vi "Read UDVs.vi"(7 "R/W Case":T1, 8 "error in (no error)":errorcluster, 9 "Output FIFO buffer in":dbl[](array[numeric]), 10 "Output Data in":T6 {"BD Refs"."Data Reference" format="%.0x"}, 11 "UDVs in":T2[](array[typedef]) {"VS ref" format="%.0x"}) -> (0 "error out":errorcluster, 1 "Output FIFO buffer out":dbl[](array[numeric]), 2 "Output Data out":T6 {"BD Refs"."Data Reference" format="%.0x"}, 3 "UDVs out":T2[](array[typedef]) {"VS ref" format="%.0x"})   [LabVIEW 2016, in "Scan Engine Custom Device.lvlib"]
uses:
  Scan Engine Custom Device.lvlib
  Type Defs/Output Data.ctl
  <vilib>/NI Veristand/Custom Device API/Block Data Reference.ctl
  <vilib>/NI Veristand/Custom Device API/Data Reference.ctl
  Type Defs/UDV Data.ctl
  <vilib>/NI Veristand/Custom Device API/Custom Device Item Ref.ctl
  Type Defs/UDV Data Type.ctl
  Type Defs/FXP Config.ctl
  Type Defs/RW Case.ctl
  <vilib>/NI Veristand/Custom Device API/Global Data Refs.vi
  <vilib>/NI Veristand/Custom Device API/Custom Device API.lvlib
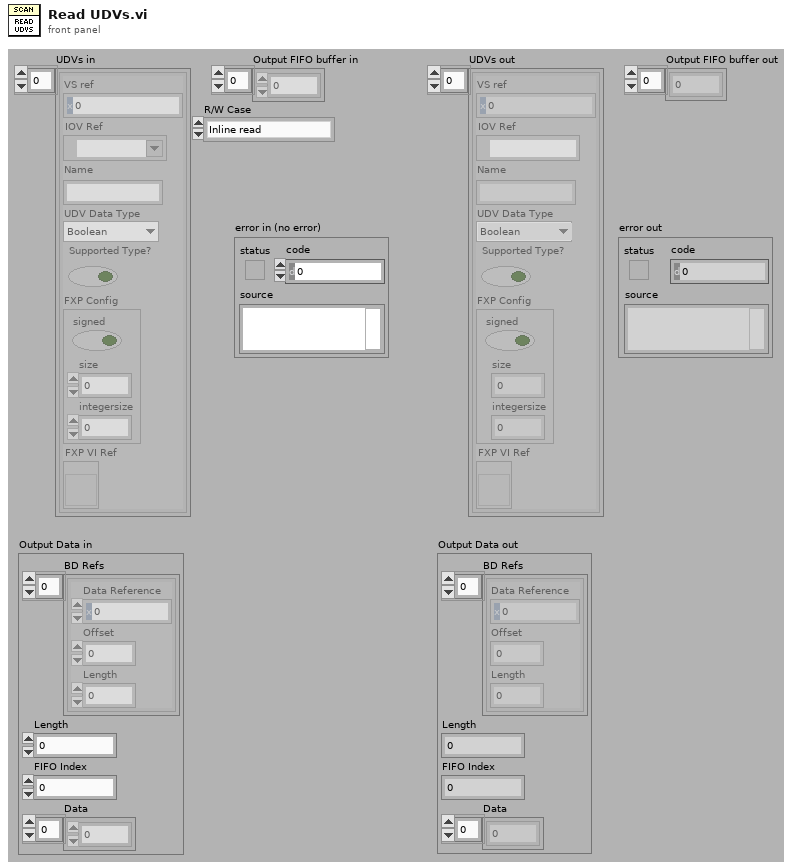
[diagram p1: front panel]
types:
  T1 = typedef "Scan Engine Custom Device.lvlib/RW Case.ctl" = enum16{"Inline read", "Inline write", "Async - Inline loop read", "Async - Inline loop write", "Async loop (read/write)"}
  T2 = typedef "Scan Engine Custom Device.lvlib/UDV Data.ctl" = cluster{"VS ref":T3, "IOV Ref":refnum<k21>, "Name":string, "UDV Data Type":T4, "Supported Type?":bool, "FXP Config":T5, "FXP VI Ref":refnum<vi>}
  T3 = typedef "Custom Device API.lvlib/Custom Device Item Ref.ctl" = u64
  T4 = typedef "Scan Engine Custom Device.lvlib/UDV Data Type.ctl" = enum16{"Boolean", "Fixed Point", "Int8", "Int16", "Int32", "Int64", "U32 Bit Field", "UInt8", "UInt16", "UInt32", "UInt64", "Other"}
  T5 = typedef "Scan Engine Custom Device.lvlib/FXP Config.ctl" = cluster{"signed":bool, "size":u32, "integersize":i32}
  T6 = typedef "Scan Engine Custom Device.lvlib/Output Data.ctl" = cluster{"BD Refs":T7[], "Length":i32, "FIFO Index":i32, "Data":dbl[]}
  T7 = typedef "Custom Device API.lvlib/Block Data Reference.ctl" = cluster{"Data Reference":T8, "Offset":u64, "Length":u64}
  T8 = typedef "Custom Device API.lvlib/Data Reference.ctl" = i32
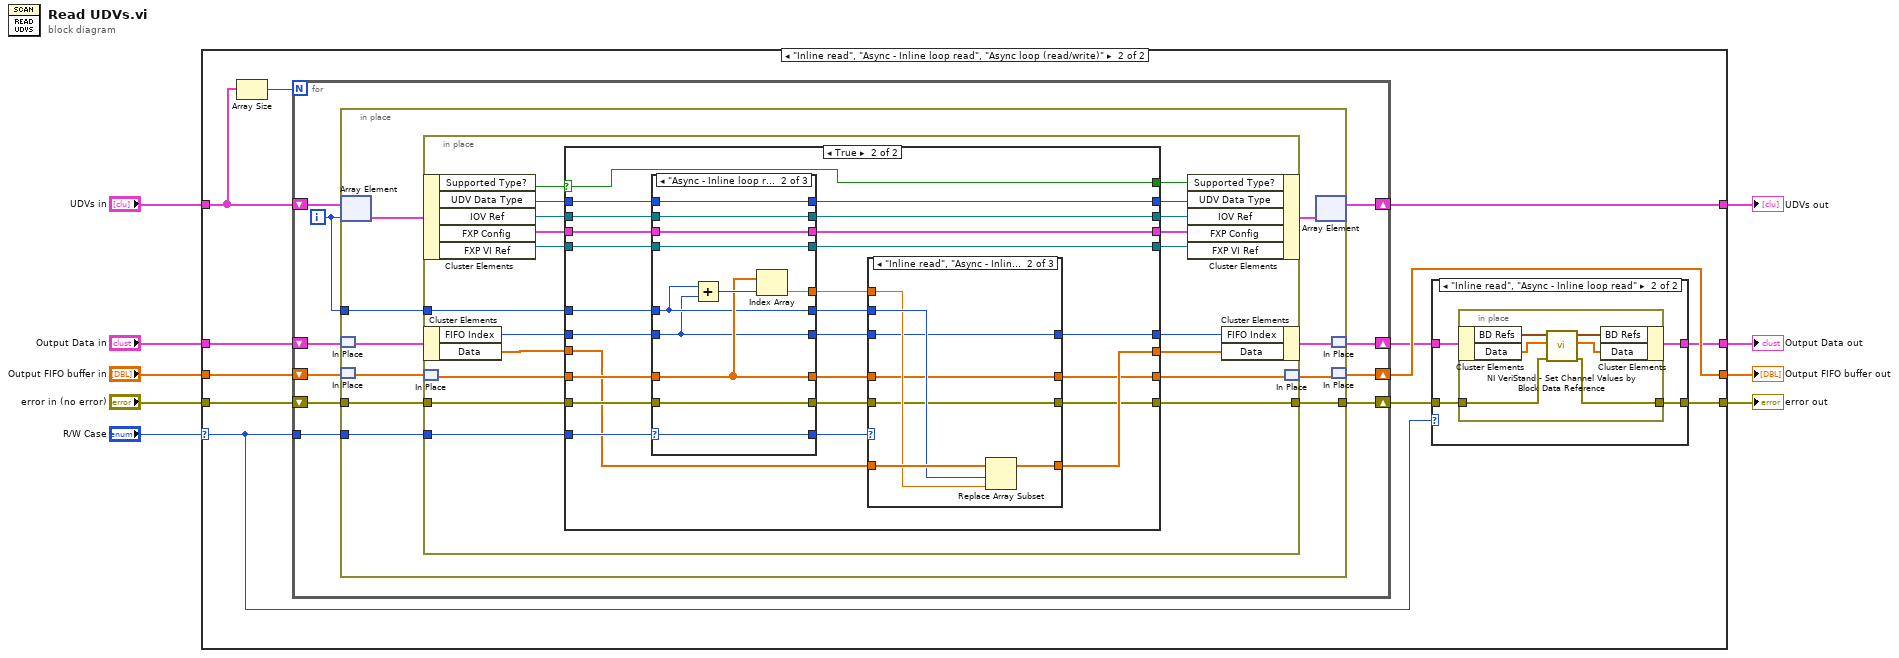
[diagram p0: block diagram]
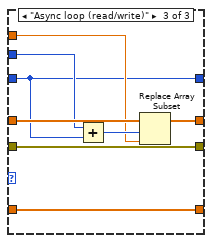
[diagram p5: hidden frame]
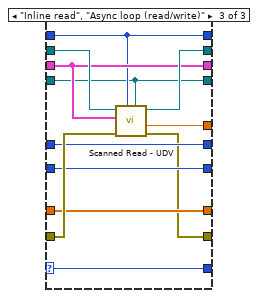
[diagram p7: hidden frame]
diagram:
  n1 = case shown="\"Inline read\", \"Async - Inline loop read\", \"Async loop (read/write)\"" "R/W Case" {
    selector: "R/W Case" -> [_ w14]
    tunnel: [w11 w25] -> w2
    tunnel: "Output FIFO buffer in" -> [w11 w24]
    tunnel: [w12 w16] -> w9
    tunnel: [w13 w23] -> w8
    tunnel: "Output Data in" -> [w12 w22]
    tunnel: "UDVs in" -> [w13 w21]
    tunnel: [w10 w15] -> w5
    tunnel: "error in (no error)" -> [w10 w19]
    frame Default {
    }
    frame "Inline read", "Async - Inline loop read", "Async loop (read/write)" {
      n2 = Array Size(array=w21) -> (size(s)=w20:i32)
      n3 = for {
        N: w20 -> [_]
        shift-right: [w34] -> w23
        shift-left: w21 -> [w35]
        shift-right: [w26] -> w18
        shift-left: w22 -> [w29]
        shift-right: [w32] -> w25
        shift-left: w24 -> [w33]
        shift-right: [w30] -> w17
        shift-left: w19 -> [w31]
        tunnel: w14 -> [w28]
        i -> [w27]
        n4 = in-place {
          in-place-border: w31 -> [w42]
          in-place-border: [w36] -> w30
          in-place-border: w28 -> [w41]
          in-place-border: w27 -> [w40]
          n5 = in-place-array #1(w35, w27) -> (w45:T2)
          n6 = in-place-match #2(w29) -> (w44:T6)
          n7 = in-place-match #3(w33) -> (w43:dbl[])
          n8 = in-place {
            in-place-border: w42 -> [w58]
            in-place-border: w41 -> [w46]
            in-place-border: w40 -> [w59]
            in-place-border: [w52] -> w36
            n9 = in-place-cluster #4(w45) -> ("Supported Type?"=w65:bool, "UDV Data Type"=w61:T4, "IOV Ref"=w60:refnum<k21>, "FXP Config"=w64:T5, "FXP VI Ref"=w63:refnum<vi>)
            n10 = in-place-cluster #5(w44) -> ("FIFO Index"=w50:i32, "Data"=w62:dbl[])
            n11 = in-place-match #6(w43) -> (w49:dbl[])
            n12 = case shown="True" w65 {
              selector: w65 -> [w73 w90]
              tunnel: w64 -> [w70 w96]
              tunnel: w63 -> [w69 w95]
              tunnel: w50 -> [w68 w94]
              tunnel: w62 -> [w67 w79]
              tunnel: w46 -> [_ w99]
              tunnel: w61 -> [w72 w98]
              tunnel: w60 -> [w71 w97]
              tunnel: w49 -> [w66 w93]
              tunnel: w59 -> [_ w92]
              tunnel: w58 -> [w74 w91]
              tunnel: [w73 w90] -> w57
              tunnel: [w72 w89] -> w56
              tunnel: [w71 w88] -> w55
              tunnel: [w70 w87] -> w54
              tunnel: [w69 w86] -> w53
              tunnel: [w74 w76] -> w52
              tunnel: [w68 w78] -> w47
              tunnel: [w67 w77] -> w51
              tunnel: [w66 w75] -> w48
              frame False {
              }
              frame True {
                n13 = case shown="\"Async - Inline loop read\"" w99 {
                  selector: w99 -> [w119 w133 w141]
                  tunnel: w98 -> [w120 w131 w142]
                  tunnel: w97 -> [w121 w132 w150]
                  tunnel: w96 -> [w122 w130 w148]
                  tunnel: w95 -> [w123 w129 w140]
                  tunnel: w94 -> [w125 w134 w145]
                  tunnel: w93 -> [w126 w137 w144]
                  tunnel: [w126 w137 w144] -> w81
                  tunnel: w92 -> [w124 w135 w146]
                  tunnel: [_ w136 w139] -> w82
                  tunnel: [w124 w135 w146] -> w84
                  tunnel: [w125 w134 w145] -> w83
                  tunnel: [w119 w133 w141] -> w85
                  tunnel: [w121 w132 w149] -> w88
                  tunnel: [w120 w131 w142] -> w89
                  tunnel: [w122 w130 w148] -> w87
                  tunnel: [w123 w129 w140] -> w86
                  tunnel: w91 -> [w127 w128 w147]
                  tunnel: [w127 w128 w143] -> w80
                  frame Default {
                  }
                  frame "Async - Inline loop read" {
                    n14 = Add(x=w135, y=w134) -> (x+y=w138:i32)
                    n15 = Index Array(array=w137, index=w138) -> (element=w136:dbl)
                  }
                  frame "Inline read", "Async loop (read/write)" {
                    n16 = call "Scanned Read - UDV.vi"("FXP VI Ref"=w140, "UDV Data Type"=w142, "error in (no error)"=w147, "FXP Config"=w148, "IOV ref in"=w150) -> ("error out"=w143:errorcluster, "data out"=w139:dbl, "IOV ref out"=w149:refnum<k21>)  [unwired: 4 in]
                  }
                }
                n17 = case shown="\"Inline read\", \"Async - Inline loop read\"" w85 {
                  tunnel: w84 -> [_ w109 w117]
                  tunnel: w83 -> [w103 w104 w111]
                  tunnel: w82 -> [_ w108 w115]
                  tunnel: w81 -> [w100 w105 w118]
                  tunnel: w80 -> [w101 w106 w113]
                  tunnel: w79 -> [w102 w110 w112]
                  tunnel: [w103 w104 w111] -> w78
                  tunnel: [w102 w107 w112] -> w77
                  tunnel: [w101 w106 w113] -> w76
                  tunnel: [w100 w105 w114] -> w75
                  frame Default {
                  }
                  frame "Inline read", "Async - Inline loop read" {
                    n18 = Replace Array Subset(array=w110, new element=w108, index=w109) -> (w107:dbl[])
                  }
                  frame "Async loop (read/write)" {
                    n19 = Add(x=w117, y=w111) -> (x+y=w116:i32)
                    n20 = Replace Array Subset(array=w118, new element=w115, index=w116) -> (w114:dbl[])
                  }
                }
              }
            }
            n21 = in-place-cluster #4("Supported Type?"=w57, "UDV Data Type"=w56, "IOV Ref"=w55, "FXP Config"=w54, "FXP VI Ref"=w53) -> (w39:T2)
            n22 = in-place-cluster #5("FIFO Index"=w47, "Data"=w51) -> (w38:T6)
            n23 = in-place-match #6(w48) -> (w37:dbl[])
          }
          n24 = in-place-array #1(w39) -> (w34:T2[])  [unwired: 1 out]
          n25 = in-place-match #2(w38) -> (w26:T6)
          n26 = in-place-match #3(w37) -> (w32:dbl[])
        }
      }
      n27 = case shown="\"Inline read\", \"Async - Inline loop read\"" w14 {
        tunnel: w18 -> [w151 w156]
        tunnel: w17 -> [w152 w155]
        tunnel: [w152 w154] -> w15
        tunnel: [w151 w153] -> w16
        frame Default {
        }
        frame "Inline read", "Async - Inline loop read" {
          n28 = in-place {
            in-place-border: w155 -> [w158]
            in-place-border: [w157] -> w154
            n29 = in-place-cluster #7(w156) -> ("BD Refs"=w162:T7[], "Data"=w160:dbl[])
            n30 = call <vilib>:"NI VeriStand - Set Channel Values by Block Data Reference.vi"("error in (no error)"=w158, "Values Array in"=w160, "Block Data Ref"=w162) -> ("error out"=w157:errorcluster, "Values Array out"=w159:dbl[], "Block Data Ref dup"=w161:T7[])  [unwired: 6 in]
            n31 = in-place-cluster #7("BD Refs"=w161, "Data"=w159) -> (w153:T6)
          }
        }
      }
    }
  }
  "Output FIFO buffer out" <- w2
  "Output Data out" <- w9
  "UDVs out" <- w8
  "error out" <- w5
